vi "Save Screenshot.vi"(8 "error in (no error)":errorcluster, 10 "Screen Shot Path":path, 11 "MSOX6004 in":refnum<class "MSOX6004.lvclass">) -> (0 "error out":errorcluster, 3 "MSOX6004 out":refnum<class "MSOX6004.lvclass">)   [LabVIEW 2018, in "MSOX6004.lvlib" / "MSOX6004.lvclass"]
doc: "This Override method is used to save a screen shot of the Oscope screen."
uses:
  MSOX6004.lvclass
  MSOX6004.lvclass/MSOX6004.ctl
  <instrlib>/Keysight InfiniiVision/Keysight InfiniiVision.lvlib
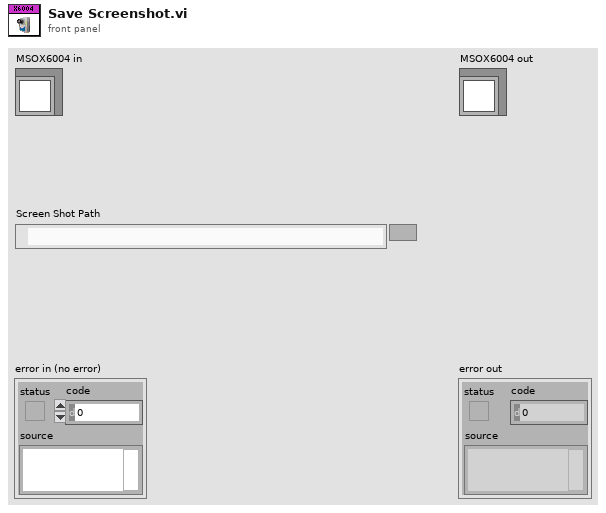
[diagram p1: front panel]
types:
  T1 = enum16{"open", "replace", "create", "open or create", "replace or create", "replace or create with confirmation"}
  T2 = typedef "MSOX6004.lvlib/MSOX6004.lvclass/Image Format.ctl" = enum16{"PNG", "BMP"}
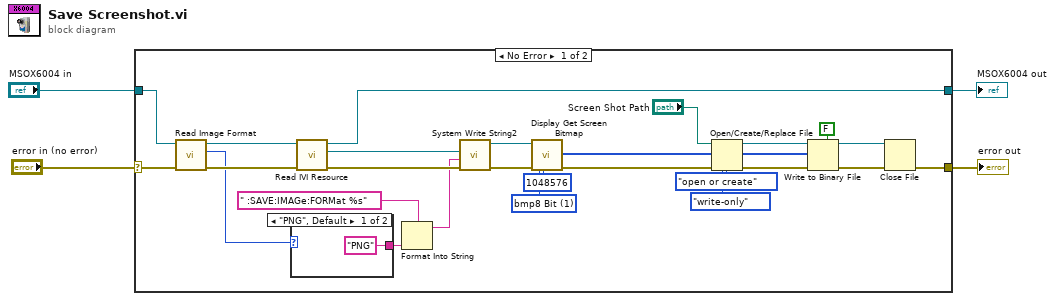
[diagram p0: block diagram]
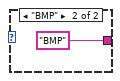
[diagram p2: hidden frame]
diagram:
  n1 = case shown="No Error" "error in (no error)" {
    selector: "error in (no error)" -> [w10 w33]
    tunnel: [w29 w34] -> w3
    tunnel: "MSOX6004 in" -> [w12 w34]
    tunnel: [w13 w33] -> w1
    frame No Error {
      w17 = 1 items=["bmp", "bmp8 Bit", "png"] ("ImageFormat (bmp)")
      n2 = call "Read Image Format.vi"("error in (no error)"=w10, "MSOX6004 in"=w12) -> ("error out"=w9:errorcluster, "Image Format"=w8:T2, "MSOX6004 out"=w11:refnum<class "MSOX6004.lvclass">)  [unwired: 7 in]
      n3 = case shown="\"PNG\", Default" w8 {
        tunnel: ["PNG" "BMP"] -> w6
        frame "PNG", Default {
        }
        frame "BMP" {
        }
      }
      n4 = call "Read IVI Resource.vi"("error in (no error)"=w9, "MSOX6004 in"=w11) -> ("error out"=w28:errorcluster, "IVI Resource"=w30:refnum<k15>, "MSOX6004 out"=w29:refnum<class "MSOX6004.lvclass">)  [unwired: 7 in]
      n5 = Format Into String(format string=" :SAVE:IMAGe:FORMat %s", w6) -> (resulting string=w5:string)  [unwired: 2 in, 1 out]
      n6 = call <instrlib>:"System Write String2.vi"("error in (no error)"=w28, "Data"=w5, "instrument handle"=w30) -> ("error out"=w15:errorcluster, "instrument handle out"=w27:refnum<k15>)  [unwired: 7 in]
      n7 = call <instrlib>:"Display Get Screen Bitmap.vi"("ValBufferSize"=1048576, "error in (no error)"=w15, "ImageFormat (bmp)"=w17, "instrument handle"=w27) -> ("error out"=w14:errorcluster, "Val"=w20:u8[])  [unwired: 4 in, 2 out]
      n8 = Open/Create/Replace File(file path (use dialog)="Screen Shot Path", error in=w14, operation (0:open)=T1."open or create", access (0:read/write)=enum16{"read/write", "read-only", "write-only"}."write-only") -> (refnum out=w23:refnum<file>, error out=w24:errorcluster)  [unwired: 2 in, 1 out]
      n9 = Write to Binary File(file (use dialog)=w23, data=w20, error in=w24, 5:FALSE ("prepend array or string size? (T)")) -> (refnum out=w25:refnum<file>, error out=w26:errorcluster)  [unwired: 2 in, 1 out]
      n10 = Close File(refnum=w25, error in=w26) -> (error out=w13:errorcluster)  [unwired: 1 out]
    }
    frame Error {
    }
  }
  "error out" <- w1
  "MSOX6004 out" <- w3
